vi "fibonacci.vi"() -> ()   [LabVIEW 2019]
panel:
  in  "Tab Control":enum32{"Fibonacci"}(tab)
  in  "MAX Value":i32
  out "Array":i32[][](array[numeric])
  in  "stop":bool
  # "n"
  # "Fn"
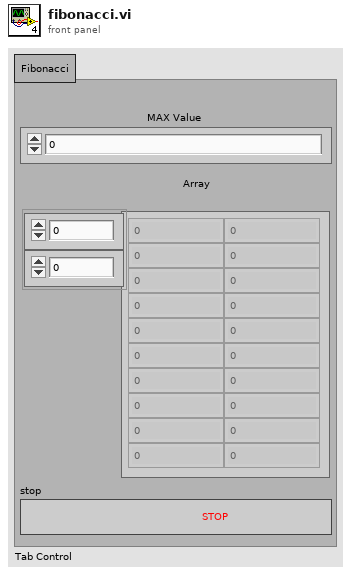
[diagram p1: front panel]
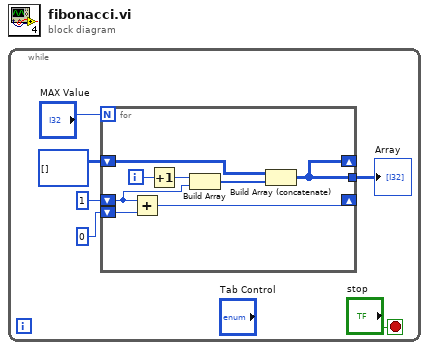
[diagram p0: block diagram]
diagram:
  n1 = while {
    stop <- "stop" stop-if-true
    n2 = for {
      N: "MAX Value" -> [_]
      shift-right: [w11] -> _
      shift-left: 1 -> [w10]
      shift-left: 0 -> [w12]
      shift-right: [w7] -> _
      shift-left: i32[][] [] -> [w8]
      tunnel: [w7] -> w1
      i -> [w14]
      n3 = Add(x=w10, y=w12) -> (x+y=w11:i32)
      n4 = Increment(x=w14) -> (x+1=w13:i32)
      n5 = Build Array(w13, w10) -> (w9:i32[])
      n6 = Build Array (concatenate)(w8, w9) -> (w7:i32[][])
    }
    "Array" <- w1
  }
